vi "App_Main Data(FGV).vi"(6 "FGV Method":T1, 8 "error in":errorcluster, 11 "Main Data In":T2={"VI Refnum"=refnum, "Subpanel"=refnum, "Connection ID"=refnum, "Meta data"=[], "Main Queue"={"Main Loop Queue"=refnum}, "User Data"={"Name"="Guset", "Email"="", "Phone Number"="", "User Picture"=array225x225[50625 elements], "Last Login Time"=timestamp(0 s since 1904-01-01)}}) -> (0 "error out":errorcluster, 3 "Main Data Out":T2={"VI Refnum"=refnum, "Subpanel"=refnum, "Connection ID"=refnum, "Meta data"=[], "Main Queue"={"Main Loop Queue"=refnum}, "User Data"={"Name"="Guset", "Email"="", "Phone Number"="", "User Picture"=array225x225[50625 elements], "Last Login Time"=timestamp(0 s since 1904-01-01)}})   [LabVIEW 2015, in "Application 2.lvlib"]
uses:
  Application 2.lvlib
  Data Def/App_Main Data.ctl
  Com VIs/Data Def/stm_MetaElement.ctl
  Com VIs/Data Def/stm_MetaDataElement.ctl
  Data Def/App_Main Queue.ctl
  Data Def/App_Main Loop Queue Data.ctl
  Com VIs/Data Def/User Data.ctl
  Data Def/App_FGV Method.ctl
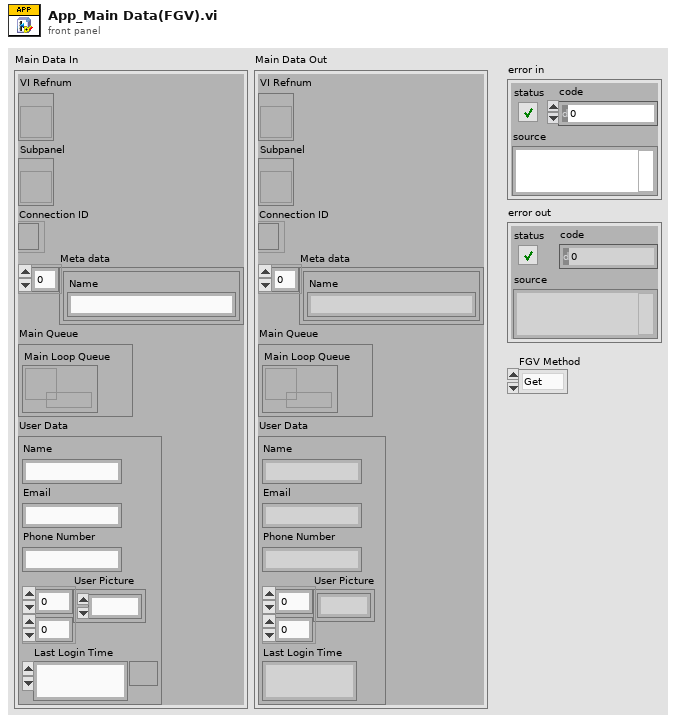
[diagram p1: front panel]
types:
  T1 = typedef "Application 2.lvlib/App_FGV Method.ctl" = enum16{"Get", "Put"}
  T2 = typedef "Application 2.lvlib/App_Main Data.ctl" = cluster{"VI Refnum":refnum<vi>, "Subpanel":refnum<vi>, "Connection ID":refnum<k5>, "Meta data":T3[], "Main Queue":T5, "User Data":T6}
  T3 = typedef "stm_MetaElement.ctl" = cluster{"Name":T4}
  T4 = typedef "stm_MetaDataElement.ctl" = string
  T5 = typedef "Application 2.lvlib/App_Main Queue.ctl" = cluster{"Main Loop Queue":refnum<queue>}
  T6 = typedef "User Data.ctl" = cluster{"Name":string, "Email":string, "Phone Number":string, "User Picture":u32[][], "Last Login Time":timestamp}
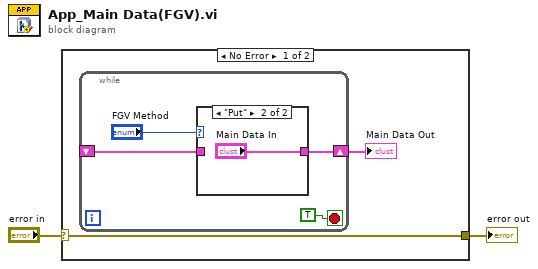
[diagram p0: block diagram]
diagram:
  n1 = case shown="No Error" "error in" {
    selector: "error in" -> [w3 w11]
    tunnel: [w3 w11] -> w1
    frame No Error {
      n2 = while {
        shift-right: [w6] -> w4
        shift-left: _ -> [w5]
        stop <- TRUE stop-if-true
        n3 = case shown="\"Put\"" "FGV Method" {
          tunnel: [w9 "Main Data In"] -> w6
          tunnel: w5 -> [w9 _]
          frame "Get", Default {
          }
          frame "Put" {
          }
        }
      }
      "Main Data Out" <- w4
    }
    frame Error {
    }
  }
  "error out" <- w1
